vi "SeCrTs-RD AI Search Channel.vi"(11 "AI Data":waveform(dbl)[](array[waveform])) -> (3 "FeedBack":dbl[](array[numeric]))   [LabVIEW 2022 SP3]
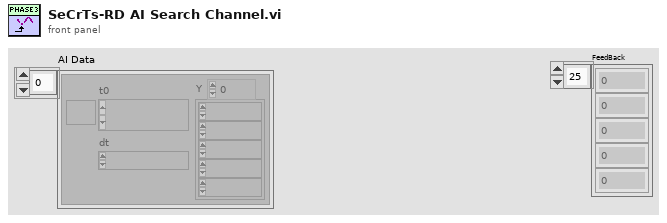
[diagram p1: front panel]
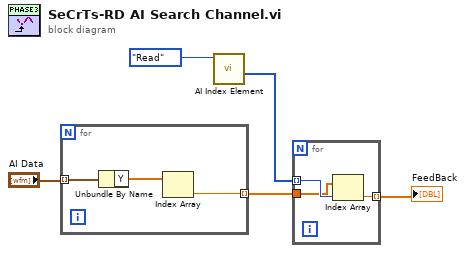
[diagram p0: block diagram]
diagram:
  n1 = for {
    tunnel: "AI Data" -> [w7] mode=indexing
    tunnel: [w6] -> w3 mode=indexing
    n2 = Unbundle By Name(w7) -> ("Y"=w8:dbl[])
    n3 = Index Array(array=w8) -> (element=w6:dbl)  [unwired: 1 in]
  }
  n4 = call "AI Index Element.vi"("Write/Read"=enum16{"Write", "Read"}."Read") -> ("Ai Index Element"=w1:i32[])  [unwired: 10 in]
  n5 = for {
    tunnel: w1 -> [w11] mode=indexing
    tunnel: w3 -> [w10]
    tunnel: [w9] -> w5 mode=indexing
    n6 = Index Array(array=w10, index=w11) -> (element=w9:dbl)
  }
  "FeedBack" <- w5
